vi "zmq_libpath.vi"(1 "path override":path) -> (0 "path":path)   [LabVIEW 2025, in "ZeroMQ.lvlib"]
doc: "Returns an absolute path to the LVZMQ shared library on the host system."
uses:
  ZeroMQ.lvlib
  <vilib>/Utility/LVLibp/NI_PackedLibraryUtility.lvlib
panel:
  # "ØMQ"
  # "labview"
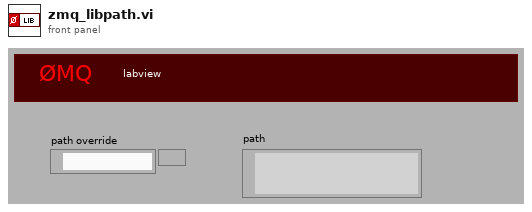
[diagram p1: front panel]
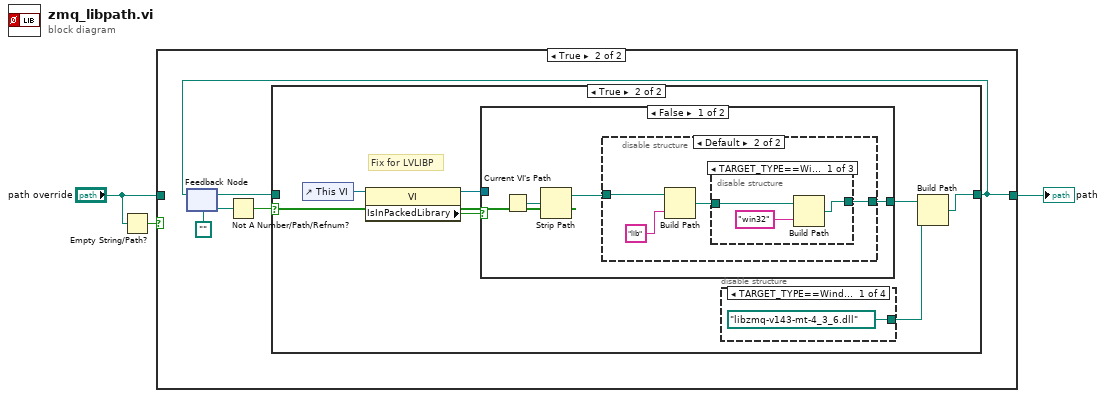
[diagram p0: block diagram]
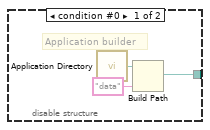
[diagram p4: hidden frame]
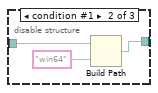
[diagram p5: hidden frame]
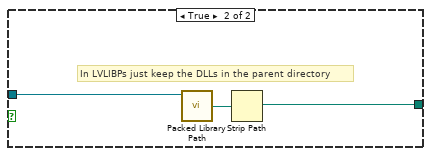
[diagram p7: hidden frame]
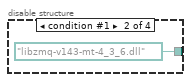
[diagram p8: hidden frame]
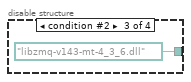
[diagram p9: hidden frame]
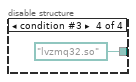
[diagram p10: hidden frame]
diagram:
  n1 = Empty String/Path?(string/path="path override") -> (empty?=w2:bool)
  n2 = case shown="True" w2 {
    tunnel: [w4 w5] -> w3
    tunnel: "path override" -> [w4 _]
    frame False {
    }
    frame True {
      n3 = feedback #1(path "") -> (w6:path)
      n4 = Not A Number/Path/Refnum?(number/path/refnum=w6) -> (NaN/Path/Refnum?=w7:bool)
      n5 = case shown="True" w7 {
        tunnel: w6 -> [w9 _]
        tunnel: [w9 w14] -> w5
        frame False {
        }
        frame True {
          # "Fix for LVLIBP"
          n6 = control-ref of="This VI"() -> (w12:refnum<vi>)
          n7 = property class="VI"(reference=w12) -> (reference out=w11:refnum<vi>, "IsInPackedLibrary"=w13:bool)  [unwired: 1 in, 1 out]
          n8 = case shown="False" w13 {
            tunnel: w11 -> [_ w35]
            tunnel: [w16 w33] -> w10
            frame False {
              n9 = Current VI's Path() -> (path=w18:path)
              n10 = Strip Path(path=w18) -> (stripped path=w17:path)  [unwired: 1 out]
              n11 = disable-structure shown="Default" {
                disable-tunnel: [w21 w25] -> w16
                disable-tunnel: w17 -> [_ w22]
                frame condition #0 {
                  # "Application builder"
                  n12 = call <vilib>:"Application Directory.vi"() -> ("Application Directory"=w19:path)
                  n13 = Build Path(base path=w19, name or relative path="data") -> (appended path=w21:path)
                }
                frame condition #1 (active) {
                  n14 = Build Path(base path=w22, name or relative path="lib") -> (appended path=w23:path)
                  n15 = disable-structure shown="TARGET_TYPE==Windows&&TARGET_BITNESS==32" {
                    disable-tunnel: [w26 w29 w32] -> w25
                    disable-tunnel: w23 -> [w27 w30 w32]
                    frame condition #0 (active) {
                      n16 = Build Path(base path=w27, name or relative path="win32") -> (appended path=w26:path)
                    }
                    frame condition #1 {
                      n17 = Build Path(base path=w30, name or relative path="win64") -> (appended path=w29:path)
                    }
                    frame condition #2 {
                    }
                  }
                }
              }
            }
            frame True {
              # "In LVLIBPs just keep the DLLs in the parent directory"
              n18 = call <vilib>:"Packed Library Path.vi"("vi reference"=w35) -> ("packed library path"=w34:path)  [unwired: 2 in, 2 out]
              n19 = Strip Path(path=w34) -> (stripped path=w33:path)  [unwired: 1 out]
            }
          }
          n20 = disable-structure shown="TARGET_TYPE==Windows&&TARGET_BITNESS==32" {
            disable-tunnel: [path "libzmq-v143-mt-4_3_6.dll" ("appended path") path "libzmq-v143-mt-4_3_6.dll" ("appended path") path "libzmq-v143-mt-4_3_6.dll" ("appended path") path "lvzmq32.so" ("appended path")] -> w15
            frame condition #0 (active) {
            }
            frame condition #1 {
            }
            frame condition #2 {
            }
            frame condition #3 {
            }
          }
          n21 = Build Path(base path=w10, name or relative path=w15) -> (appended path=w14:path)
        }
      }
      n22 = feedback-in #1(w5) -> ()
    }
  }
  "path" <- w3
